vi "TutorialGenerateDisplay.vi"() -> ()   [LabVIEW 2010]
doc: "该模板用于生成信号，并在图中显示。可结合《LabVIEW入门手册》中的练习使用该模板。\n注:在本模板的VI中，默认情况下LabVIEW将启用自动错误处理。"
uses:
  Instance           1 33Saved   TutorialGenerateDisplay 2 .vi
  Instance           2 33Saved   TutorialGenerateDisplay 2 .vi
panel:
  out "最小值":dbl
  out "最大值":dbl
  out "算术平均":dbl
  in  "滑动杆":dbl(slide) scale=0.0..10.0
  out "Waveform Graph":dynamicdata(graph) caption="波形图"
  in  "stop":bool caption="停止"
  # "生成和显示信号"
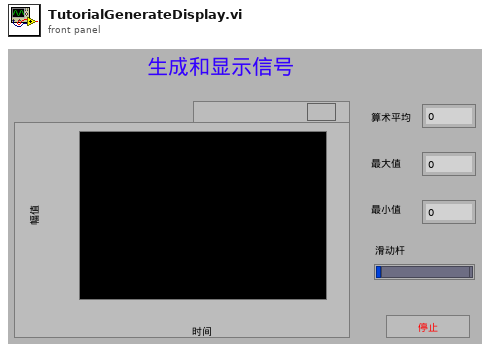
[diagram p1: front panel]
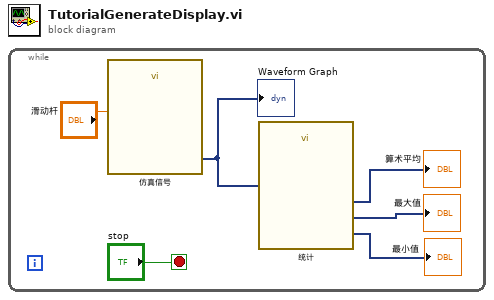
[diagram p0: block diagram]
diagram:
  n1 = while {
    stop <- "stop" stop-if-true
    n2 = call "仿真信号"("噪声幅值"="滑动杆") -> ("三角与均匀噪声"=w4:dynamicdata)  [unwired: 13 in, 1 out]
    "Waveform Graph" <- w4
    n3 = call "统计"("Signals"=w4) -> ("Arithmetic Mean"=→"算术平均":dynamicdata, "Minimum"=→"最小值":dynamicdata, "Maximum"=→"最大值":dynamicdata)  [unwired: 23 in, 1 out]
  }
